vi "Vision Research Phantom Series PhFile PhSetUseCase.vi"(0 "CH [in]":u32, 1 "CineUseCaseID [in]":T1 items=["UC_VIEW"=1, "UC_SAVE"=2], 5 "Error In (no error)":errorcluster) -> (14 "hC [out]":u32, 19 "Error Out":errorcluster)   [LabVIEW 2013, in "VRI.lvlib"]
doc: "PhSetUseCase\nHRESULT PhSetUseCase(CINEHANDLE CH, int CineUseCaseID);\n\nParameters\nCH [in]\n Cine to set the use case for.\ncineUseCaseID [in]\n Desired use case. Possible values are:\n UC_VIEW: Images requested from this cine are going to be displayed/played\n UC_SAVE: Images requested from this cine are going to be written to file\n\nReturn Value\nThe function returns ERR_Ok in case of success or an error code, otherwise. To get extended error information call PhGetErrorMessage.\n\nRemarks\nA cine use case tells how this cine will be used and it mainly refers to cine images use. One can request cine images in order to save them to file or it can request cine images in order to display them in a video player application. Different processing steps and different optimizations apply in each of these situations. The use case represents a simple way of hiding all of these details.\nBy default, each cine has its use case set to UC_VIEW.\nPlease note that a cine (a CINEHANDLE object) cannot have more than one use case set at a time. When needing to display and save images from the same cine in parallel create one CINEHANDLE for each situation and set a corresponding use case for each of them.\n\nRequired Header\nPhFile.h"
uses:
  VRI.lvlib
  _Type Defs/PhFile CineUseCaseID.ctl
  Phantom DLLs/PhFile.Dll
panel:
  # "For instructions on the use of this VI, press Ctrl+H to display the help window and move the mouse over the icon, controls, and indicators"
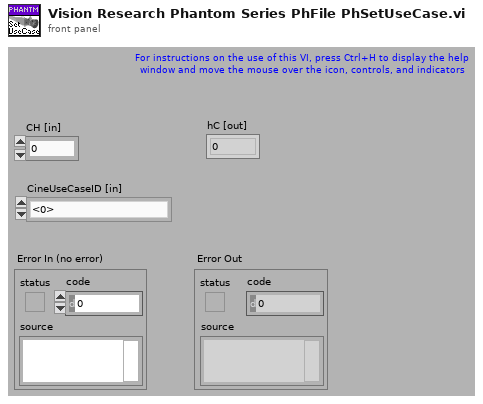
[diagram p1: front panel]
types:
  T1 = typedef "VRI.lvlib/PhFile CineUseCaseID.ctl" = u16
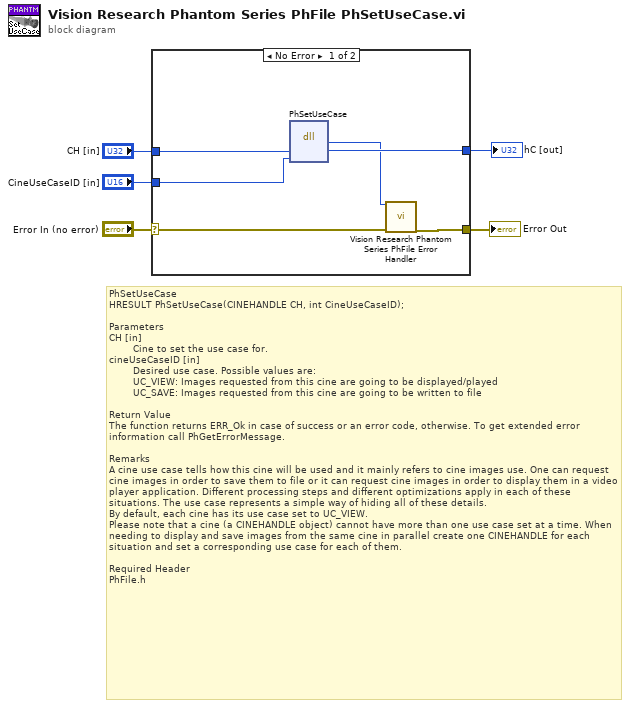
[diagram p0: block diagram]
diagram:
  # "PhSetUseCase\nHRESULT PhSetUseCase(CINEHANDLE CH, int CineUseCaseID);\n\nParameters\nCH [in]\n\t       Cine to set the use case for.\ncineUseCaseID [in]\n\t\t      Desired use case. Possible values are:\n\t       UC_VIEW: Images requested from this cine are going to be displayed/played\n\t       UC_SAVE: Images requested from this cine are going to be written to file\n\nReturn Value\nThe function returns ERR_Ok in case of success or an error code, otherwise. To get extended error information call PhGetErrorMessage.\n\nRemarks\nA cine use case tells how this cine will be used and it mainly refers to cine images use. One can request cine images in order to save them to file or it can request cine images in order to display them in a video player application. Different processing steps and different optimizations apply in each of these situations. The use case represents a simple way of hiding all of these details.\nBy default, each cine has its use case set to UC_VIEW.\nPlease note that a cine (a CINEHANDLE object) cannot have more than one use case set at a time. When needing to display and save images from the same cine in parallel create one CINEHANDLE for each situation and set a corresponding use case for each of them.\n\nRequired Header\nPhFile.h"
  n1 = case shown="No Error" "Error In (no error)" {
    selector: "Error In (no error)" -> [w11 w13]
    tunnel: [w10 w13] -> w4
    tunnel: "CH [in]" -> [w9 w12]
    tunnel: "CineUseCaseID [in]" -> [w8 _]
    tunnel: [w7 w12] -> w1
    frame No Error {
      n2 = dll-call lib="C:/Projects/SDK/64-bit/Vision Research Phantom Series Labview Driver/Phantom DLLs/PhFile.dll" fn="PhSetUseCase"("hC"=w9, "CineUseCaseID"=w8) -> ("HRESULT"=w6:i32, "hC"=w7:u32)  [unwired: 3 in, 3 out]
      n3 = call "Vision Research Phantom Series PhFile Error Handler.vi"("Error Code (0)"=w6, "Error In (no error)"=w11) -> ("Error Out"=w10:errorcluster)  [unwired: 17 out]
    }
    frame Error {
    }
  }
  "Error Out" <- w4
  "hC [out]" <- w1
